vi "Read CD Template.vi"(8 "error in (no error)":errorcluster, 11 "NIVS_Consolidated_CDW_MetaDataObj in":refnum<class "NIVS_Consolidated_CDW_MetaDataObj.lvclass">) -> (0 "error out":errorcluster, 2 "CD Template":refnum<class "NIVS_CD Template.lvclass">, 3 "NIVS_Consolidated_CDW_MetaDataObj out":refnum<class "NIVS_Consolidated_CDW_MetaDataObj.lvclass">)   [LabVIEW 2020, in "NIVS_Consolidated_CDW_MetaDataObj.lvclass"]
uses:
  NIVS_Consolidated_CDW_MetaDataObj.lvclass
  Template Classes/NIVS_CD Template/NIVS_CD Template.lvclass
  NIVS_Consolidated_CDW_MetaDataObj.lvclass/NIVS_Consolidated_CDW_MetaDataObj.ctl
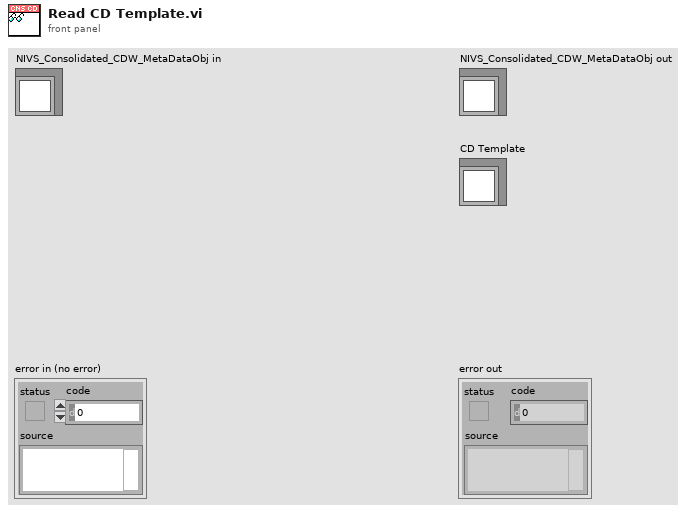
[diagram p1: front panel]
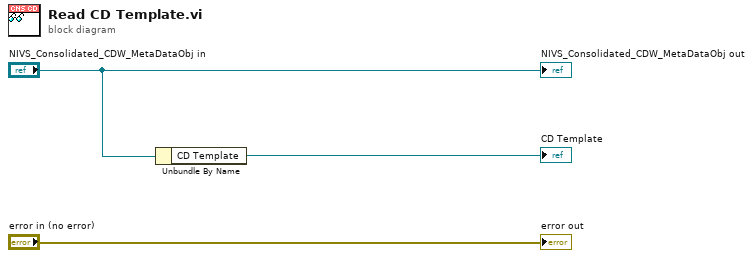
[diagram p0: block diagram]
diagram:
  n1 = Unbundle By Name("NIVS_Consolidated_CDW_MetaDataObj in") -> ("CD Template"=→"CD Template":refnum<class "NIVS_CD Template.lvclass">)
  "error out" <- "error in (no error)"
  "NIVS_Consolidated_CDW_MetaDataObj out" <- "NIVS_Consolidated_CDW_MetaDataObj in"
